vi "Degrees to Radians.vi"(1 "Degrees IN":dbl) -> (0 "Radians OUT":dbl)   [LabVIEW 2015]
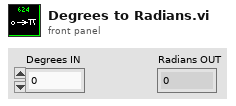
[diagram p1: front panel]
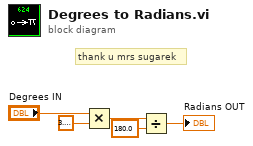
[diagram p0: block diagram]
diagram:
  # "thank u mrs sugarek"
  n1 = Multiply(x="Degrees IN", y=3.141592653589793) -> (x*y=w3:dbl)
  n2 = Divide(x=w3, y=180.0) -> (x/y=→"Radians OUT":dbl)
